vi "lvlibp_install.vi"(6 "lvlib_move_directory":path, 8 "error in (no error)":errorcluster, 11 "build_specifications":T1) -> (0 "error out":errorcluster)   [LabVIEW 2015, in "lv-builder.lvlib"]
uses:
  lv-builder.lvlib
  lv-build/public/_controls/build_specification.ctl
  lv-build/public/_controls/build_type.ctl
  <vilib>/Utility/error.llb/Error Cluster From Error Code.vi
  <vilib>/ErrorRing/Error Ring.xnode
  lv-build/lv-build.lvlib
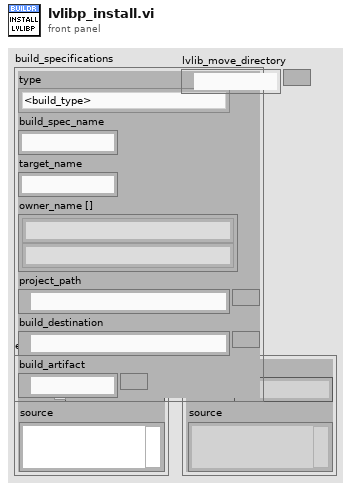
[diagram p1: front panel]
types:
  T1 = typedef "lv-build.lvlib/build_specification.ctl" = cluster{"type":T2, "build_spec_name":string, "target_name":string, "owner_name []":string[], "project_path":path, "build_destination":path, "build_artifact":path}
  T2 = typedef "lv-build.lvlib/build_type.ctl" = enum16{"<build_type>", "application_pc", "application_rt", "installer", "llb", "lvlibp", "zip", "fpga", "<null>"}
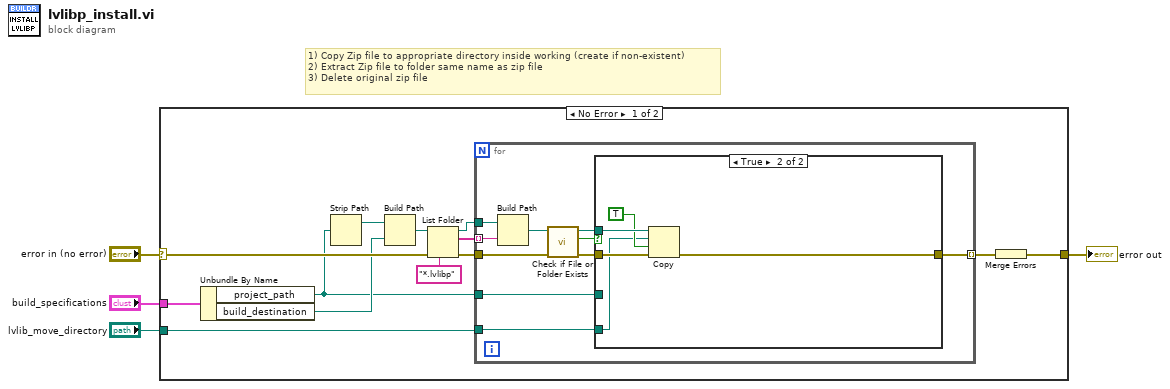
[diagram p0: block diagram]
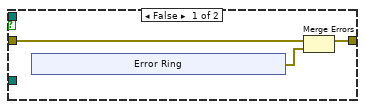
[diagram p2: hidden frame]
diagram:
  # "1) Copy Zip file to appropriate directory inside working (create if non-existent)\n2) Extract Zip file to folder same name as zip file\n3) Delete original zip file"
  n1 = case shown="No Error" "error in (no error)" {
    selector: "error in (no error)" -> [w15 w40]
    tunnel: "build_specifications" -> [w17 _]
    tunnel: [w10 w40] -> w3
    tunnel: "lvlib_move_directory" -> [w5 _]
    frame No Error {
      n2 = Unbundle By Name(w17) -> ("project_path"=w6:path, "build_destination"=w8:path)
      n3 = Strip Path(path=w6) -> (stripped path=w7:path)  [unwired: 1 out]
      n4 = Build Path(base path=w7, name or relative path=w8) -> (appended path=w9:path)
      n5 = List Folder(path=w9, pattern="*.lvlibp", error in=w15) -> (path out=w13:path, filenames=w14:string[], error out=w12:errorcluster)  [unwired: 1 in, 1 out]
      n6 = for {
        tunnel: w14 -> [w27] mode=indexing
        tunnel: w13 -> [w26]
        tunnel: w6 -> [w20]
        tunnel: w12 -> [w24]
        tunnel: [w22] -> w11 mode=indexing
        tunnel: w5 -> [w18]
        n7 = Build Path(base path=w26, name or relative path=w27) -> (appended path=w25:path)
        n8 = call <vilib>:"Check if File or Folder Exists.vi"("error in (no error)"=w24, "path"=w25) -> ("error out"=w23:errorcluster, "file or folder exists?"=w19:bool, "dup path"=w21:path)  [unwired: 7 in]
        n9 = case shown="True" w19 {
          tunnel: w23 -> [w28 w38]
          tunnel: [w29 w36] -> w22
          tunnel: w21 -> [_ w39]
          tunnel: w20 -> [_ _]
          tunnel: w18 -> [_ w35]
          frame False {
            n10 = xnode "Error Ring"() -> ("error out"=w30:errorcluster)
            n11 = Merge Errors(w28, w30) -> (w29:errorcluster)
          }
          frame True {
            n12 = Copy(8:w38, 9:TRUE ("overwrite (F)"), 10:w35, 11:w39) -> (0:w36:errorcluster)  [unwired: 1 in, 2 out]
          }
        }
      }
      n13 = Merge Errors(w11) -> (w10:errorcluster)
    }
    frame Error {
    }
  }
  "error out" <- w3
